vi "get Wait For Response.vi"(8 "error in (no error)":errorcluster, 11 "REx Command - Root in":refnum<class "REx Command - Root.lvclass">) -> (0 "error out":errorcluster, 2 "Wait For Response? (T)":bool=TRUE, 3 "REx Command - Root out":refnum<class "REx Command - Root.lvclass">)   [LabVIEW 2012, in "REx.lvlib" / "REx Command - Root.lvclass"]
uses:
  REx Command - Root.lvclass
  REx Command - Root.lvclass/REx Command - Root.ctl
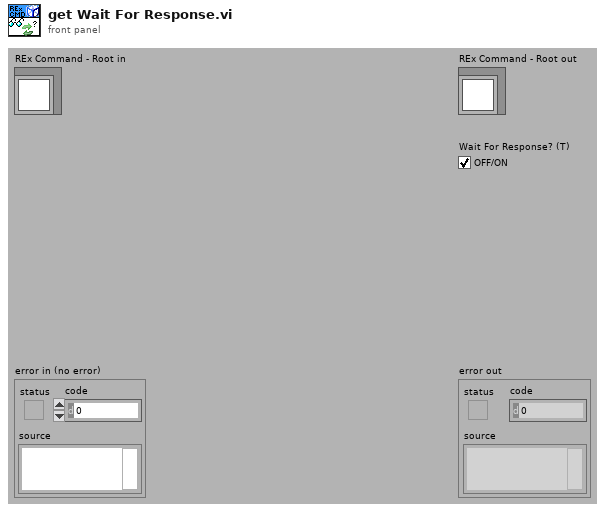
[diagram p1: front panel]
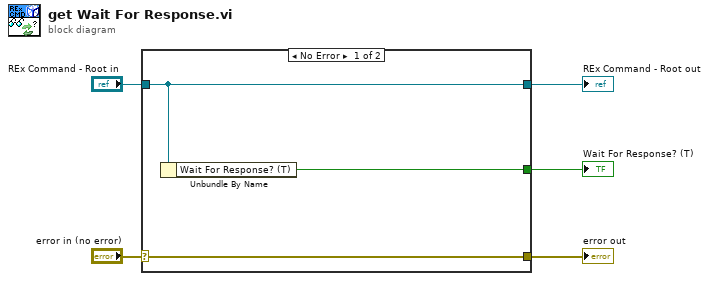
[diagram p0: block diagram]
diagram:
  n1 = case shown="No Error" "error in (no error)" {
    selector: "error in (no error)" -> [w8 w9]
    tunnel: [w8 w9] -> w4
    tunnel: [w7 w10] -> w2
    tunnel: "REx Command - Root in" -> [w7 w10]
    tunnel: [w6 _] -> w1
    frame No Error {
      n2 = Unbundle By Name(w7) -> ("Wait For Response? (T)"=w6:bool)
    }
    frame Error {
    }
  }
  "error out" <- w4
  "REx Command - Root out" <- w2
  "Wait For Response? (T)" <- w1
